vi "PKG_IMC_GetNetCardName.vi"(10 "name":string, 11 "index":i32) -> (2 "name out":string, 3 "function return":i32)   [LabVIEW 2018, in "IMC_Pkg4xxx.lvlib"]
doc: "PKG_IMC_GetNetCardName (int index, char name[256]);"
uses:
  IMC_Pkg4xxx.lvlib
  IMC_Pkg4xxx.dll
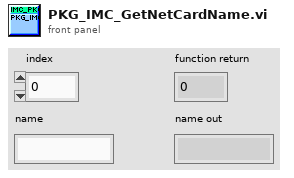
[diagram p1: front panel]
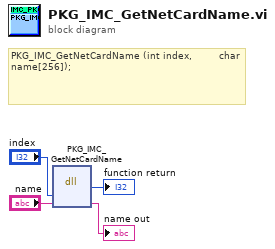
[diagram p0: block diagram]
diagram:
  # "PKG_IMC_GetNetCardName (int index,\t\t\t\t\t\t\t\t\tchar name[256]);"
  n1 = dll-call lib="PTH2\\abs D做的项目航天测量驱动电机IMCAppincLabview32\nIMC_Pkg4xxx.*" fn="PKG_IMC_GetNetCardName"("index"="index", "name"="name") -> (→"function return":i32, "name"=→"name out":string)  [unwired: 4 in, 2 out]
